vi "Add User Defined Message.vi"(8 "error in (no error)":errorcluster, 11 "Node Ptr":u64 format="%.0x") -> (0 "error out":errorcluster)   [LabVIEW 2015, in "Diagnostics Addon System Explorer.lvlib"]
uses:
  Diagnostics Addon System Explorer.lvlib
  Types/FG.Action.ctl
  Shared/Types/Type.ctl
  <vilib>/NI Veristand/Custom Device API/Custom Device Channel.ctl
  <vilib>/NI Veristand/Custom Device API/Custom Device Channel Type.ctl
  Shared/SubVIs/Constants.vi
  <vilib>/NI/NIVS System Definition Utilities/SysDef API/SysDef.Property.Set.vi
  <vilib>/NI/NIVS System Definition Utilities/_SubVIs/SysDef.Property.Set.U32.vi
  <vilib>/NI Veristand/Custom Device API/NI VeriStand - Get Item Property.vi
  <vilib>/NI Veristand/Custom Device API/Get Item Property (U32).vi
  Shared/Diagnostics Addon Shared.lvlib
  <vilib>/NI VeriStand/Custom Device API/Custom Device API.lvlib
panel:
  in  "Tag":string
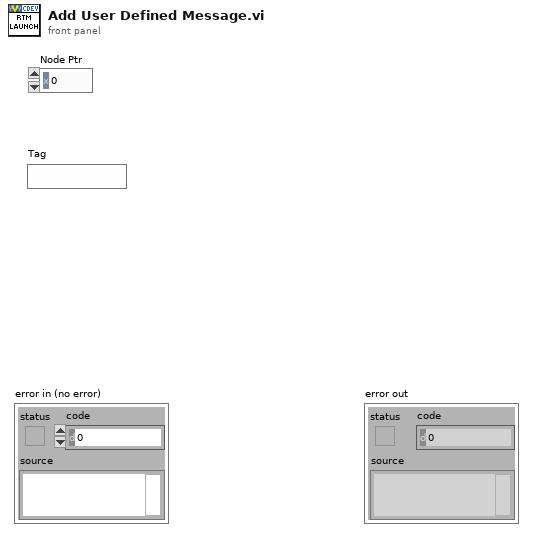
[diagram p1: front panel]
types:
  T1 = typedef "Custom Device API.lvlib/Custom Device Channel.ctl" = cluster{"Type":T2, "Units":string, "Default Value":dbl, "Faultable":bool, "Scalable":bool}
  T2 = typedef "Custom Device API.lvlib/Custom Device Channel Type.ctl" = enum16{"Input", "Output"}
  T3 = typedef "Diagnostics Addon Shared.lvlib/Type.ctl" = enum16{"DID", "CDID", "PID", "CPID", "Read Memory", "Write Memory", "DTC Control", "IO Cmd", "IO Resp", "Routine Start Cmd", "Routine Start Resp", "Routine Request Cmd", "Routine Request Resp", "Routine Stop Cmd", "Routine Stop Resp", "UserDefined Cmd", "UserDefined Rsp"}
  T4 = typedef "Diagnostics Addon System Explorer.lvlib/FG.Action.ctl" = enum16{"Get", "Set"}
  T5 = typedef "Custom Device API.lvlib/Custom Device Item Ref.ctl" = u64
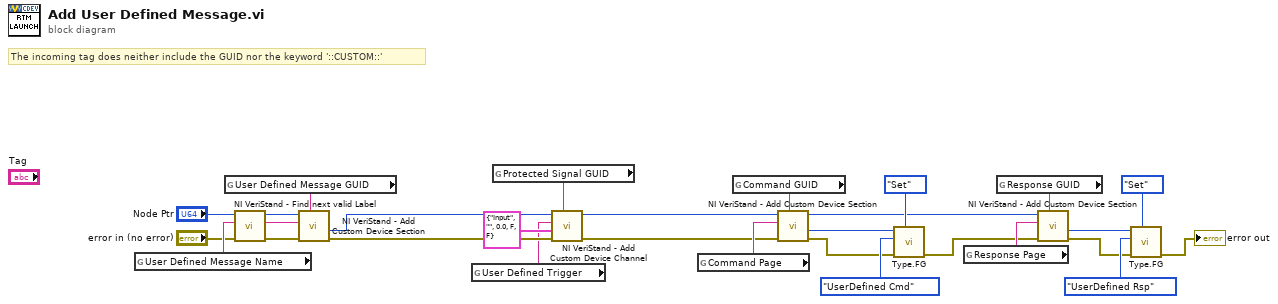
[diagram p0: block diagram]
diagram:
  # "The incoming tag does neither include the GUID nor the keyword '::CUSTOM::'"
  n1 = global read "Constants.vi" "User Defined Message Name"() -> (w27:string)
  n2 = global read "Constants.vi" "User Defined Message GUID"() -> (w29:string)
  n3 = call <vilib>:"NI VeriStand - Find next valid Label.vi"("error in (no error)"="error in (no error)", "Label"=w27, "Item Ref in"="Node Ptr") -> ("error out"=w26:errorcluster, "Label out"=w25:string, "Item Ref out"=w28:T5)  [unwired: 4 in, 2 out]
  n4 = call <vilib>:"NI VeriStand - Add Custom Device Section.vi"("GUID (Default Section)"=w29, "error in (no error)"=w26, "Section Name"=w25, "Parent Ref in"=w28) -> ("error out"=w5:errorcluster, "Section Ptr"=w3:T5)  [unwired: 4 in, 2 out]
  n5 = global read "Constants.vi" "User Defined Trigger"() -> (w1:string)
  n6 = global read "Constants.vi" "Protected Signal GUID"() -> (w6:string)
  n7 = call <vilib>:"NI VeriStand - Add Custom Device Channel.vi"("GUID (Default Channel)"=w6, "error in (no error)"=w5, "Channel"=T1 {"Type"=enum."Input", "Units"="", "Default Value"=0.0, "Faultable"=FALSE, "Scalable"=FALSE}, "Channel Name"=w1, "Parent Ref in"=w3) -> ("error out"=w4:errorcluster, "Parent Ref out"=w2:T5)  [unwired: 3 in, 2 out]
  n8 = global read "Constants.vi" "Command Page"() -> (w22:string)
  n9 = global read "Constants.vi" "Command GUID"() -> (w21:string)
  n10 = call <vilib>:"NI VeriStand - Add Custom Device Section.vi"("GUID (Default Section)"=w21, "error in (no error)"=w4, "Section Name"=w22, "Parent Ref in"=w2) -> ("error out"=w14:errorcluster, "Section Ptr"=w13:T5, "Parent Ref out"=w11:T5)  [unwired: 4 in, 1 out]
  n11 = call "Type.FG.vi"("Action"=FG.Action."Set", "error in (no error)"=w14, "Type"=Type."UserDefined Cmd", "Device Item Ref in"=w13) -> ("error out"=w12:errorcluster)  [unwired: 5 in, 2 out]
  n12 = global read "Constants.vi" "Response Page"() -> (w19:string)
  n13 = global read "Constants.vi" "Response GUID"() -> (w20:string)
  n14 = call <vilib>:"NI VeriStand - Add Custom Device Section.vi"("GUID (Default Section)"=w20, "error in (no error)"=w12, "Section Name"=w19, "Parent Ref in"=w11) -> ("error out"=w10:errorcluster, "Section Ptr"=w9:T5)  [unwired: 4 in, 2 out]
  n15 = call "Type.FG.vi"("Action"=FG.Action."Set", "error in (no error)"=w10, "Type"=Type."UserDefined Rsp", "Device Item Ref in"=w9) -> ("error out"=→"error out":errorcluster)  [unwired: 5 in, 2 out]
